vi "Error Global.vi"() -> ()   [LabVIEW 2025, in "I2C Bus Monitor UI.lvlib"]
uses:
  I2C Bus Monitor UI.lvlib
panel:
  out "Startup Note":string="I2C Bus Monitor Plugin\n\nNOTE\n\nIf you would like to use this plugin in parallel with another session using the same FPGA resource, \nmake sure of the following: \n\n1. In your parallel session, you must use one of the bitfiles that corresponds to your device model from this directory:\n\n\"C:\\Program Files\\NI\\LVAddons\\flexrioii\\1\\ProjectTemplates\\Source\\FlexRIO\\NI148X\\Getting Started\\FPGA Bitfiles\"\n\nFor example, if you are using \"PXIe-1486 (4In 4Out)\" module, it would be the following bitfile:\n\n\"C:\\Program Files\\NI\\LVAddons\\flexrioii\\1\\ProjectTemplates\\Source\\FlexRIO\\NI148X\\Getting Started\\FPGA Bitfiles\\PXIe_1486_4_In_4_Out_Acq_Tap.lvbitx\"\n\n2. In your parallel session, make sure you are NOT accessing the \"User Timestamps\" FIFO, because it is used by this plugin to monitor the I2C bus traffic. "
  out "-7051":string="<b>No Serial Inputs on this Device</b>\n\nSpecified Resource Name:\n%s\n\nSpecified Model:\n%s"
  out "-7050":string="<b>Unsupported Device</b>\n\nSpecified Resource Name:\n%s\n\nSpecified Model :\n%s\n\nSupported Models:\n%s"
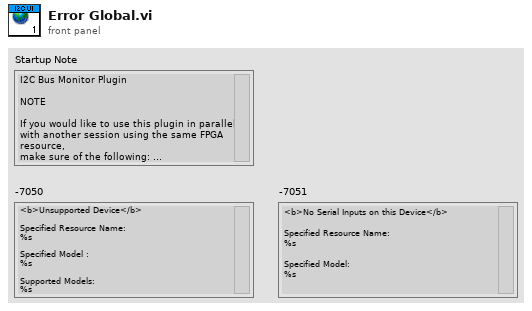
[diagram p1: front panel]
diagram:
